vi "Get Text in Bookmark.vi"(8 "error in (no error)":errorcluster, 10 "String":string, 11 "Word_Report in":refnum<class "Word_Report.lvclass">) -> (0 "error out":errorcluster, 1 "found":bool, 2 "Text":string, 3 "Word_Report out":refnum<class "Word_Report.lvclass">)   [LabVIEW 2018, in "WordReportGeneration.lvlib" / "Word_Report.lvclass"]
uses:
  Word_Report.lvclass
  C:/Program Files (x86)/National Instruments/LabVIEW 2018/vi.lib/Utility/NIReport.llb/NI_report.lvclass
  <vilib>/Utility/NIReport.llb/Word/NI_Word.lvclass
  WordReportGeneration.lvlib
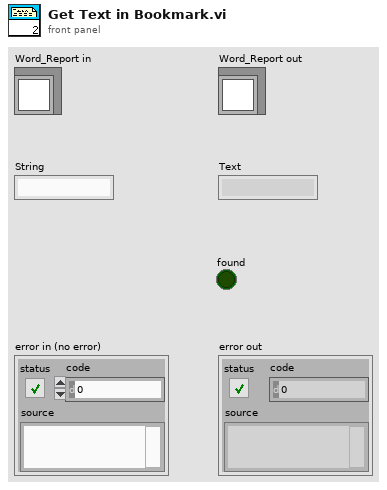
[diagram p1: front panel]
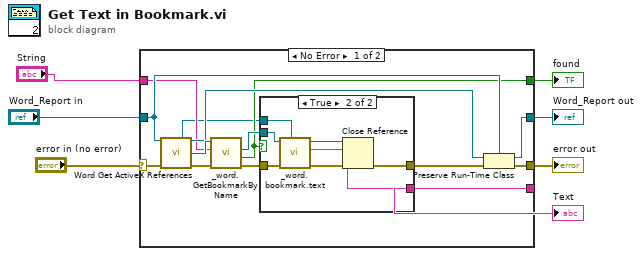
[diagram p0: block diagram]
diagram:
  n1 = case shown="No Error" "error in (no error)" {
    selector: "error in (no error)" -> [w20 w30]
    tunnel: [w18 _] -> w6
    tunnel: [w14 w31] -> w5
    tunnel: "Word_Report in" -> [w13 w31]
    tunnel: [w12 w30] -> w3
    tunnel: [w11 _] -> w2
    tunnel: "String" -> [w10 _]
    frame No Error {
      n2 = call <vilib>:"Word Get ActiveX References.vi"("report in"=w13, "error in (no error)"=w20) -> ("Word._Application"=w9:refnum<k7>, "report out"=w15:refnum<class "NI_report.lvclass">, "Word._Document"=w16:refnum<k7>, "error out"=w21:errorcluster)  [unwired: 7 in, 3 out]
      n3 = call "_word.GetBookmarkByName.vi"("error in (no error)"=w21, "String"=w10, "Document"=w16) -> ("error out"=w19:errorcluster, "found"=w11:bool, "bookmark"=w17:refnum<k7>)  [unwired: 5 in, 1 out]
      n4 = case shown="True" w11 {
        tunnel: w19 -> [w22 w29]
        tunnel: [_ w28] -> w18
        tunnel: w17 -> [_ w27]
        tunnel: w9 -> [_ w26]
        tunnel: [w22 w24] -> w8
        frame False {
        }
        frame True {
          n5 = call "_word.bookmark.text.vi"("Application"=w26, "error IO"=w29, "Bookmark"=w27) -> ("error out"=w25:errorcluster, "Text"=w28:string, "Bookmark(dup)"=w23:refnum<k7>)  [unwired: 6 in]
          n6 = Close Reference(reference=w23, error in (no error)=w25) -> (error out=w24:errorcluster)
        }
      }
      n7 = Preserve Run-Time Class(object in=w15, error in=w8, 2:w13) -> (object out=w14:refnum<class "Word_Report.lvclass">, error out=w12:errorcluster)
    }
    frame Error {
    }
  }
  "error out" <- w3
  "Text" <- w6
  "Word_Report out" <- w5
  "found" <- w2
